vi "DistractMostProbableValueFromImage-1.vi"(7 "[IN] # Iteration":i32, 8 "error in":errorcluster, 11 "[IN] Max Projected Image":T1) -> (0 "error out":errorcluster, 3 "[OUT] Processed Image":T1, 5 "[OUT] # Iteration":i32)   [LabVIEW 2020]
doc: "Draws the cross for showing a center of mass"
uses:
  <vilib>/vision/Image Controls.llb/IMAQ Image.ctl
  <vilib>/vision/NI_Vision_Development_Module.lvlib
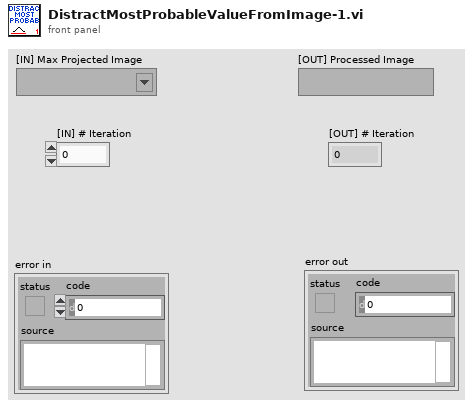
[diagram p1: front panel]
types:
  T1 = typedef "IMAQ Image.ctl" = refnum<image>
  T2 = cluster{"histogram":u32[], "Minimal Value":sgl, "Maximal Value":sgl, "Starting Value":sgl, "Interval Width":sgl, "Mean Value":sgl, "Standard  Variation":sgl, "Area (pixels)":i32}
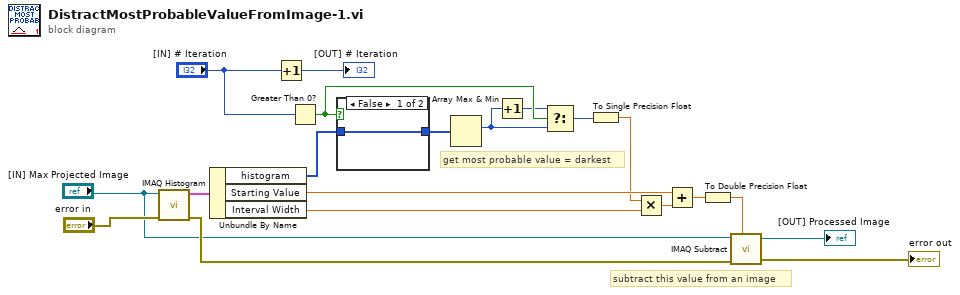
[diagram p0: block diagram]
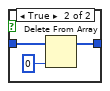
[diagram p2: hidden frame]
diagram:
  # "subtract this value from an image"
  # "get most probable value = darkest"
  n1 = call "IMAQ Histogram"("error in (no error)"="error in", "Image"="[IN] Max Projected Image") -> ("error out"=w14:errorcluster, "Histogram Report"=w19:T2)  [unwired: 8 in]
  n2 = Unbundle By Name(w19) -> ("histogram"=w8:u32[], "Starting Value"=w18:sgl, "Interval Width"=w16:sgl)
  n3 = Increment(x="[IN] # Iteration") -> (x+1=→"[OUT] # Iteration":i32)
  n4 = Greater Than 0?(x="[IN] # Iteration") -> (x > 0?=w6:bool)
  n5 = case shown="False" w6 {
    tunnel: w8 -> [w21 w23]
    tunnel: [w21 w22] -> w7
    frame False {
    }
    frame True {
      n6 = Delete From Array(array=w23, index=0) -> (array with subset deleted=w22:u32[])  [unwired: 1 in, 1 out]
    }
  }
  n7 = Array Max & Min(array=w7) -> (max index (indices)=w4:i32)  [unwired: 3 out]
  n8 = Increment(x=w4) -> (x+1=w3:i32)
  n9 = Select(t=w3, s=w6, f=w4) -> (s? t:f=w5:i32)
  n10 = To Single Precision Float(number=w5) -> (single precision float=w17:sgl)
  n11 = Multiply(x=w17, y=w16) -> (x*y=w15:sgl)
  n12 = Add(x=w18, y=w15) -> (x+y=w2:sgl)
  n13 = To Double Precision Float(number=w2) -> (double precision float=w1:dbl)
  n14 = call "IMAQ Subtract"("Image Src A"="[IN] Max Projected Image", "Constant"=w1, "error in (no error)"=w14) -> ("Image Dst Out"=→"[OUT] Processed Image":T1, "error out"=→"error out":errorcluster)  [unwired: 4 in]
